vi "breakfast menu sub vi.vi"() -> ()   [LabVIEW 2019]
uses:
  Program Files (x86)/National Instruments/LabVIEW 2019/project/EN1Course-master (12)/EN1Course-master/_Subs/ThingWorx/_TW_Subs/TW_XControl.xctl
  Program Files (x86)/National Instruments/LabVIEW 2019/project/EN1Course-master (12)/EN1Course-master/_Subs/ThingWorx/_TW_Subs/Thingworx_Write_string.vi
  Program Files (x86)/National Instruments/LabVIEW 2019/project/EN1Course-master (12)/EN1Course-master/_Subs/ThingWorx/_TW_Subs/Thingworx_Write_Bool.vi
panel:
  in  "Bread":string(xcontrol)="Day1:MadBB"
  in  "B MEAT":string(xcontrol)="Day1:MadBM"
  in  "B POT":string(xcontrol)="Day1:MadBP"
  in  "BENTREE 2":string(xcontrol)="Day1:MadBE2"
  in  "BENTREE 1":string(xcontrol)="Day1:MadBE1"
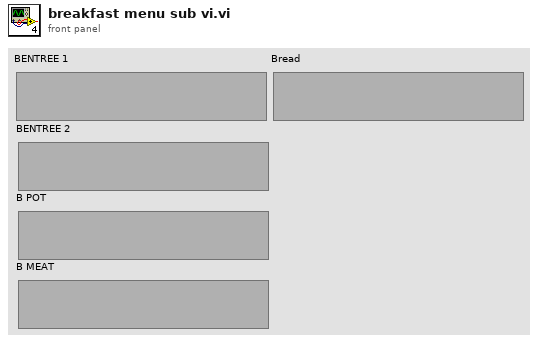
[diagram p1: front panel]
types:
  T1 = cluster{"menu-id":string, "data":cluster{"Breakfast":cluster{"BREAKFAST ENTREE":string[], "BREAKFAST POTATO":string[], "BREAKFAST MEATS":string[], "BRK BREADS,PASTRIES & TOPPINGS":string[]}}}
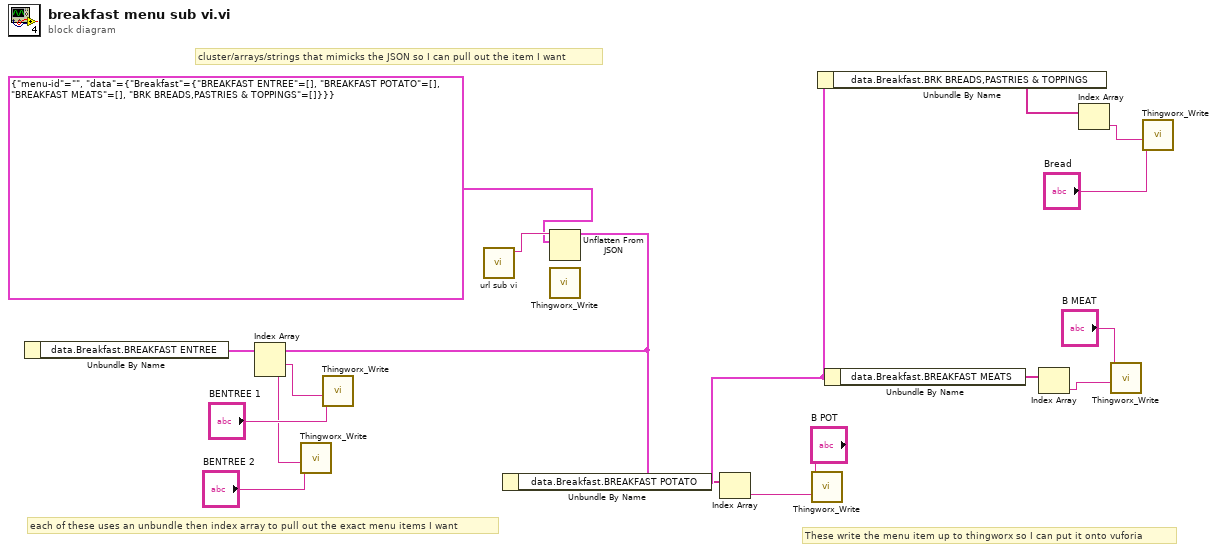
[diagram p0: block diagram]
diagram:
  # "These write the menu item up to thingworx so I can put it onto vuforia"
  # "each of these uses an unbundle then index array to pull out the exact menu items I want"
  # "cluster/arrays/strings that mimicks the JSON so I can pull out the item I want"
  n1 = call "url sub vi.vi"() -> ("body 2"=w17:string)  [unwired: 11 in]
  n2 = Unflatten From JSON(JSON string=w17, type and defaults=T1 {"menu-id"="", "data"={"Breakfast"={"BREAKFAST ENTREE"=[], "BREAKFAST POTATO"=[], "BREAKFAST MEATS"=[], "BRK BREADS,PASTRIES & TOPPINGS"=[]}}}) -> (value=w16:T1)  [unwired: 5 in, 1 out]
  n3 = Unbundle By Name(w16) -> ("data.Breakfast.BREAKFAST ENTREE"=w12:string[])
  n4 = Index Array(array=w12) -> (element #1=w10:string, element #2=w8:string)  [unwired: 2 in]
  n5 = call-poly "Thingworx_Write.vi"("String"=w8, "Thingworx"="BENTREE 2") -> ()  [unwired: 10 in]
  n6 = call-poly "Thingworx_Write.vi"("String"=w10, "Thingworx"="BENTREE 1") -> ()  [unwired: 10 in]
  n7 = Unbundle By Name(w16) -> ("data.Breakfast.BREAKFAST POTATO"=w13:string[])
  n8 = call-poly "Thingworx_Write.vi"() -> ()  [unwired: 12 in]
  n9 = Index Array(array=w13) -> (element=w6:string)  [unwired: 1 in]
  n10 = call-poly "Thingworx_Write.vi"("String"=w6, "Thingworx"="B POT") -> ()  [unwired: 10 in]
  n11 = Unbundle By Name(w16) -> ("data.Breakfast.BRK BREADS,PASTRIES & TOPPINGS"=w15:string[])
  n12 = Unbundle By Name(w16) -> ("data.Breakfast.BREAKFAST MEATS"=w14:string[])
  n13 = Index Array(array=w14) -> (element=w4:string)  [unwired: 1 in]
  n14 = Index Array(array=w15) -> (element=w2:string)  [unwired: 1 in]
  n15 = call-poly "Thingworx_Write.vi"("String"=w4, "Thingworx"="B MEAT") -> ()  [unwired: 10 in]
  n16 = call-poly "Thingworx_Write.vi"("String"=w2, "Thingworx"="Bread") -> ()  [unwired: 10 in]
